vi "lowpass.vi"(0 "MS":dbl, 2 "Boolean":bool, 3 "TC":dbl, 4 "IC Value":dbl, 5 "In":dbl) -> (1 "Out":dbl)   [LabVIEW 2025]
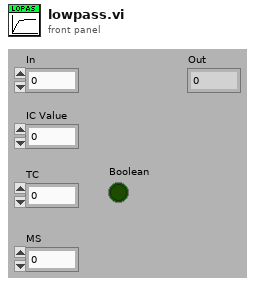
[diagram p1: front panel]
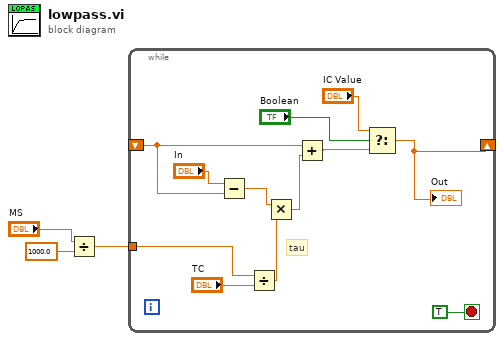
[diagram p0: block diagram]
diagram:
  n1 = Divide(x="MS", y=1000.0) -> (x/y=w1:dbl)
  n2 = while {
    shift-right: [w7] -> _
    shift-left: _ -> [w11]
    tunnel: w1 -> [w4]
    stop <- TRUE stop-if-true
    # "tau"
    n3 = Subtract(x="In", y=w11) -> (x-y=w12:dbl)
    n4 = Divide(x=w4, y="TC") -> (x/y=w9:dbl)
    n5 = Multiply(x=w12, y=w9) -> (x*y=w14:dbl)
    n6 = Add(x=w11, y=w14) -> (x+y=w8:dbl)
    n7 = Select(t="IC Value", s="Boolean", f=w8) -> (s? t:f=w7:dbl)
    "Out" <- w7
  }
